vi "Camera.vi"(0 "Camera in":refnum<class "Camera.lvclass">, 1 "Machine Vision":T4, 2 "Material":T3, 3 "Loop 0":bool, 5 "Stop":bool, 9 "BCG Image Processing":T2={"Brightness"=128.0, "Contrast"=45.0, "Gamma"=1.0} {"Brightness" scale=0.0..400.0; "Contrast" scale=0.0..90.0; "Gamma" scale=0.005..5.0}, 11 "error in (no error)":errorcluster, 12 "Camera settings":T1={"Gamma"=1.0, "Gain"=7, "Sharpness"=0, "Contrast"=0.009999999999999995, "Exposure"=0.0004073180282999787} {"Exposure" min=0.000244140625 max=0.5 scale=0.0002..0.5; "Contrast" min=0.0 max=1.0 scale=0.001..1.0; "Sharpness" min=0 max=2 step=1 scale=0.0..2.0; "Gain" min=0 max=100 step=1 scale=0.1..100.0; "Gamma" min=0.01 max=10.0 scale=0.01..10.0}, 14 "Override presets":bool) -> (4 "Camera out":refnum<class "Camera.lvclass">, 6 "Average Strength":dbl, 8 "Image":T5(plugin-control), 10 "Camera":dbl[](array[numeric]), 13 "Radius (Real-World)":dbl, 15 "error out":errorcluster)   [LabVIEW 2020, in "Camera.lvclass"]
uses:
  Camera.lvclass
  Machine Vision.ctl
  Material.ctl
  Image processing.ctl
  Camera settings.ctl
  <vilib>/vision/NI_Vision_Development_Module.lvlib
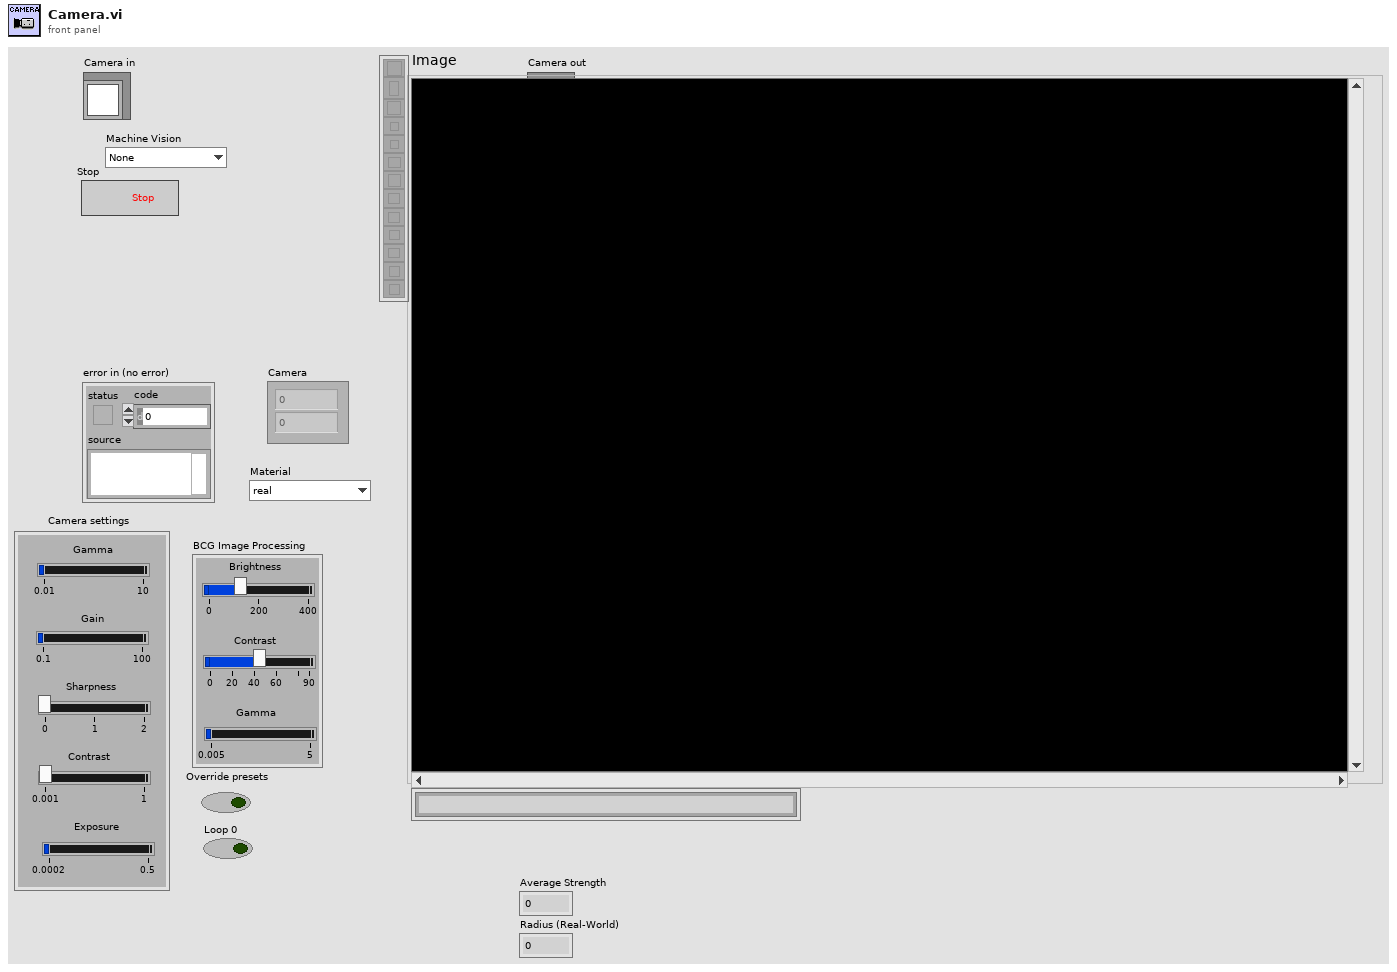
[diagram p1: front panel]
types:
  T1 = typedef "Camera.lvclass/Camera settings.ctl" = cluster{"Gamma":dbl, "Gain":i64, "Sharpness":i64, "Contrast":dbl, "Exposure":dbl}
  T2 = typedef "Camera.lvclass/Image processing.ctl" = cluster{"Brightness":sgl, "Contrast":sgl, "Gamma":sgl}
  T3 = typedef "Camera.lvclass/Material.ctl" = enum16{"real", "dummy", "PETG"}
  T4 = typedef "Camera.lvclass/Machine Vision.ctl" = enum16{"None", "Tray Fiducials", "HPK Silicon", "100um dot", "Hexaboard", "Corner (TL, BR)", "Corner (BL, TR)"}
  T5 = typedef "IMAQ Image.ctl" = refnum<image>
  T6 = cluster{"Center (Pixels)":cluster{"X":sgl, "Y":sgl}, "Radius (Pixels)":dbl, "Center (Real-World)":cluster{"X":sgl, "Y":sgl}, "Radius (Real-World)":dbl, "Roundness (Real-World)":dbl, "Average Strength":dbl, "Average SNR (dB)":dbl}
  T7 = cluster{"output string":sgl, "output string":sgl}
  T8 = typedef "ROI Descriptor" = cluster{"Global Rectangle":i32[], "Contours":cluster{"ID":enum32{"External", "Internal"}, "Type":u32, "Coordinates":i32[]}[]}
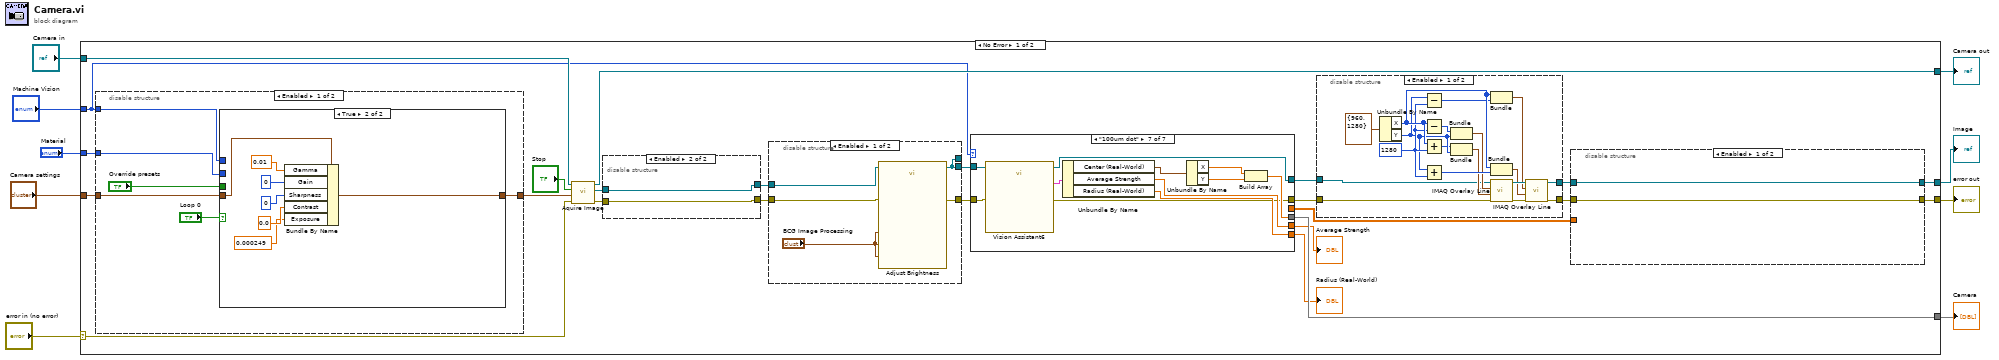
[diagram p0: block diagram]
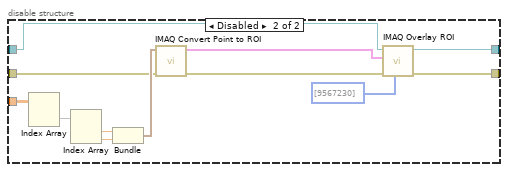
[diagram p2: hidden frame]
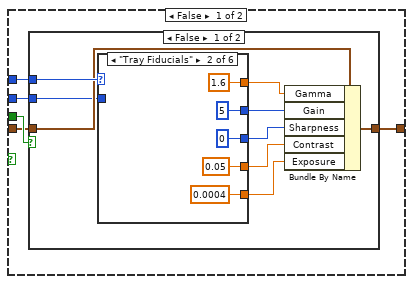
[diagram p5: hidden frame]
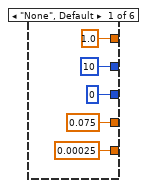
[diagram p6: hidden frame]
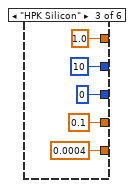
[diagram p7: hidden frame]
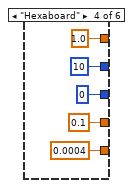
[diagram p8: hidden frame]
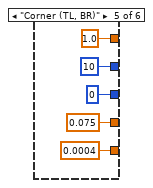
[diagram p9: hidden frame]
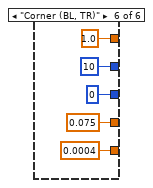
[diagram p10: hidden frame]
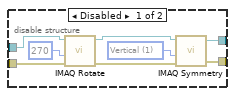
[diagram p13: hidden frame]
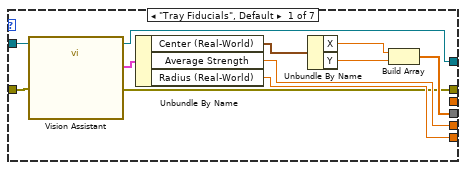
[diagram p14: hidden frame]
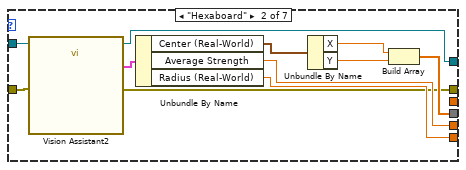
[diagram p15: hidden frame]
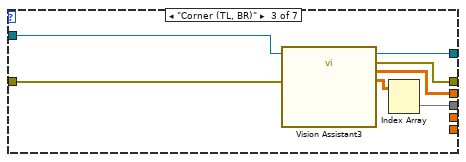
[diagram p16: hidden frame]
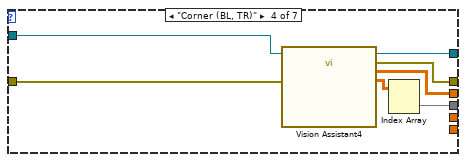
[diagram p17: hidden frame]
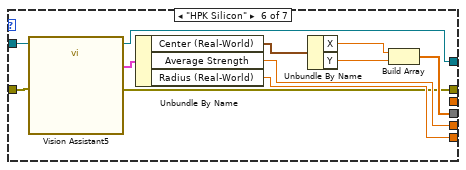
[diagram p19: hidden frame]
diagram:
  n1 = case shown="No Error" "error in (no error)" {
    selector: "error in (no error)" -> [w16 w205]
    tunnel: [w10 w205] -> w8
    tunnel: [w31 w204] -> w7
    tunnel: "Camera in" -> [w32 w204]
    tunnel: [w30 _] -> w5
    tunnel: [w20 _] -> w4
    tunnel: "Machine Vision" -> [w26 _]
    tunnel: "Camera settings" -> [w27 _]
    tunnel: "Material" -> [w25 _]
    frame No Error {
      n2 = disable-structure shown="Enabled" {
        disable-tunnel: w26 -> [w80 _]
        disable-tunnel: w27 -> [w79 w133]
        disable-tunnel: [w78 w133] -> w28
        disable-tunnel: w25 -> [w75 _]
        frame Enabled {
          n3 = case shown="True" "Loop 0" {
            tunnel: "Override presets" -> [w85 _]
            tunnel: w80 -> [w84 _]
            tunnel: w79 -> [w83 w132]
            tunnel: [w82 w131] -> w78
            tunnel: w75 -> [w81 _]
            frame False {
              n4 = case shown="False" w85 {
                tunnel: w84 -> [w94 _]
                tunnel: w83 -> [w93 w125]
                tunnel: [w87 w125] -> w82
                tunnel: w81 -> [w86 _]
                frame False {
                  n5 = case shown="\"Tray Fiducials\"" w94 {
                    tunnel: [1.0 ("Gamma::Value") 1.6 ("Gamma::Value") 1.0 ("Gamma::Value") 1.0 ("Gamma::Value") 1.0 ("Gamma::Value") 1.0 ("Gamma::Value")] -> w92
                    tunnel: [i64 10 ("Gain::Value") i64 5 ("Gain::Value") i64 10 ("Gain::Value") i64 10 ("Gain::Value") i64 10 ("Gain::Value") i64 10 ("Gain::Value")] -> w91
                    tunnel: [i64 0 ("Sharpness::Value") i64 0 ("Sharpness::Value") i64 0 ("Sharpness::Value") i64 0 ("Sharpness::Value") i64 0 ("Sharpness::Value") i64 0 ("Sharpness::Value")] -> w90
                    tunnel: [0.075 ("Contrast::Value") 0.05 ("Contrast::Value") 0.1 ("Contrast::Value") 0.1 ("Contrast::Value") 0.075 ("Contrast::Value") 0.075 ("Contrast::Value")] -> w89
                    tunnel: [0.00025 ("Exposure::Value") 0.0004 ("Exposure::Value") 0.0004 ("Exposure::Value") 0.0004 ("Exposure::Value") 0.0004 ("Exposure::Value") 0.0004 ("Exposure::Value")] -> w88
                    tunnel: w86 -> [_ _ _ _ _ _]
                    frame "None", Default {
                    }
                    frame "Tray Fiducials" {
                    }
                    frame "HPK Silicon" {
                    }
                    frame "Hexaboard" {
                    }
                    frame "Corner (TL, BR)" {
                    }
                    frame "Corner (BL, TR)" {
                    }
                  }
                  n6 = Bundle By Name(cluster=w93, "Gamma"=w92, "Gain"=w91, "Sharpness"=w90, "Contrast"=w89, "Exposure"=w88) -> (w87:T1)
                }
                frame True {
                }
              }
            }
            frame True {
              n7 = Bundle By Name(cluster=w132, "Gamma"=0.01, "Gain"=i64 0, "Sharpness"=i64 0, "Contrast"=0.0, "Exposure"=0.000249) -> (w131:T1)
            }
          }
        }
        frame Disabled {
        }
      }
      n8 = call-dynamic "Aquire Image.vi"("error in (no error)"=w16, "Cluster"=w28, "Stop"="Stop", "Camera in"=w32) -> ("error out"=w15:errorcluster, "Image Out"=w29:T5, "Camera out"=w31:refnum<class "Camera.lvclass">)  [unwired: 5 in]
      n9 = disable-structure shown="Enabled" {
        disable-tunnel: w29 -> [w140 w143]
        disable-tunnel: [w139 w143] -> w24
        disable-tunnel: w15 -> [w136 w142]
        disable-tunnel: [w134 w142] -> w14
        frame Disabled {
          w138 = u32 1 items=["Horizontal", "Vertical", "Central", "1st Diagonal", "2nd Diagonal"] ("Type of Symmetry")
          n10 = call "IMAQ Rotate"("error in (no error)"=w136, "Angle (degrees)"=270, "Image Src"=w140) -> ("error out"=w135:errorcluster, "Image Dst Out"=w137:T5)  [unwired: 7 in]
          n11 = call "IMAQ Symmetry"("error in (no error)"=w135, "Type of Symmetry"=w138, "Image Src"=w137) -> ("error out"=w134:errorcluster, "Image Dst Out"=w139:T5)  [unwired: 2 in]
        }
        frame Enabled {
        }
      }
      n12 = disable-structure shown="Enabled" {
        disable-tunnel: w24 -> [w72 w74]
        disable-tunnel: [w70 w74] -> _
        disable-tunnel: [w70 _] -> w23
        disable-tunnel: w14 -> [w69 w73]
        disable-tunnel: [w68 w73] -> w13
        frame Enabled {
          n13 = call "Adjust Brightness"("Image In"=w72, "Red BCG Values (Brightness 1)"="BCG Image Processing", "Green BCG Values (Brightness 1)"="BCG Image Processing", "Blue BCG Values (Brightness 1)"="BCG Image Processing", "error in"=w69) -> ("Image Out"=w70:T5, "error out"=w68:errorcluster)  [unwired: 21 in]
        }
        frame Disabled {
        }
      }
      n14 = case shown="\"100um dot\"" w26 {
        tunnel: [w148 w160 w170 w177 _ w188 w199] -> w30
        tunnel: [w150 w161 w172 w179 w181 w189 w200] -> w22
        tunnel: w23 -> [w151 w159 w169 w176 w181 w186 w197]
        tunnel: [w146 w157 _ _ _ w185 w196] -> w19
        tunnel: [w147 w158 _ _ _ w184 w195] -> w18
        tunnel: [_ _ w168 w175 _ _ _] -> w17
        tunnel: w13 -> [w145 w155 w167 w174 w180 w183 w194]
        tunnel: [w144 w156 w166 w173 w180 w182 w193] -> w12
        frame "Tray Fiducials", Default {
          n15 = call "Vision Assistant"("Image In"=w151, "error in"=w145) -> ("Image Out"=w150:T5, "Fitted Circle (Find Circular Edge 1)"=w149:T6, "error out"=w144:errorcluster)  [unwired: 23 in]
          n16 = Unbundle By Name(w149) -> ("Center (Real-World)"=w152:cluster{"X":sgl, "Y":sgl}, "Average Strength"=w147:dbl, "Radius (Real-World)"=w146:dbl)
          n17 = Unbundle By Name(w152) -> ("X"=w154:sgl, "Y"=w153:sgl)
          n18 = Build Array(w154, w153) -> (w148:sgl[])
        }
        frame "Hexaboard" {
          n19 = call "Vision Assistant2"("Image In"=w159, "error in"=w155) -> ("Image Out"=w161:T5, "Fitted Circle (Find Circular Edge 1)"=w163:T6, "error out"=w156:errorcluster)  [unwired: 23 in]
          n20 = Unbundle By Name(w163) -> ("Center (Real-World)"=w165:cluster{"X":sgl, "Y":sgl}, "Average Strength"=w158:dbl, "Radius (Real-World)"=w157:dbl)
          n21 = Unbundle By Name(w165) -> ("X"=w164:sgl, "Y"=w162:sgl)
          n22 = Build Array(w164, w162) -> (w160:sgl[])
        }
        frame "Corner (TL, BR)" {
          n23 = call "Vision Assistant3"("Image In"=w169, "error in"=w167) -> ("Image Out"=w172:T5, "error out"=w166:errorcluster, "Caliper Results (Top Left, Bottom Right)"=w168:sgl[][], "Calibrated Results (Top Left, Bottom Right)"=w171:sgl[][])  [unwired: 22 in]
          n24 = Index Array(array=w171) -> (element=w170:sgl[])  [unwired: 2 in]
        }
        frame "Corner (BL, TR)" {
          n25 = call "Vision Assistant4"("Image In"=w176, "error in"=w174) -> ("Image Out"=w179:T5, "error out"=w173:errorcluster, "Caliper Results (Bottom Left, Top Right)"=w175:sgl[][], "Calibrated Results (Bottom Left, Top Right)"=w178:sgl[][])  [unwired: 22 in]
          n26 = Index Array(array=w178) -> (element=w177:sgl[])  [unwired: 2 in]
        }
        frame "None" {
        }
        frame "HPK Silicon" {
          n27 = call "Vision Assistant5"("Image In"=w186, "error in"=w183) -> ("Image Out"=w189:T5, "Fitted Circle (Find Circular Edge 1)"=w187:T6, "error out"=w182:errorcluster)  [unwired: 23 in]
          n28 = Unbundle By Name(w187) -> ("Center (Real-World)"=w192:cluster{"X":sgl, "Y":sgl}, "Average Strength"=w184:dbl, "Radius (Real-World)"=w185:dbl)
          n29 = Unbundle By Name(w192) -> ("X"=w191:sgl, "Y"=w190:sgl)
          n30 = Build Array(w191, w190) -> (w188:sgl[])
        }
        frame "100um dot" {
          n31 = call "Vision Assistant6"("Image In"=w197, "error in"=w194) -> ("Image Out"=w200:T5, "Fitted Circle (Find Circular Edge 1)"=w198:T6, "error out"=w193:errorcluster)  [unwired: 23 in]
          n32 = Unbundle By Name(w198) -> ("Center (Real-World)"=w203:cluster{"X":sgl, "Y":sgl}, "Average Strength"=w195:dbl, "Radius (Real-World)"=w196:dbl)
          n33 = Unbundle By Name(w203) -> ("X"=w202:sgl, "Y"=w201:sgl)
          n34 = Build Array(w202, w201) -> (w199:sgl[])
        }
      }
      "Radius (Real-World)" <- w19
      "Average Strength" <- w18
      n35 = disable-structure shown="Enabled" {
        disable-tunnel: w22 -> [w52 w67]
        disable-tunnel: [w51 w67] -> w21
        disable-tunnel: w12 -> [w50 w66]
        disable-tunnel: [w48 w66] -> w11
        frame Enabled {
          w59 = 1280
          n36 = Unbundle By Name(cluster{"X":i32, "Y":i32} {"X"=960, "Y"=1280} ("Cross Hair coordinates")) -> ("X"=w62:i32, "Y"=w58:i32)
          n37 = Subtract(x=w58, y=w59) -> (x-y=w60:i32)
          n38 = Subtract(x=w62, y=w59) -> (x-y=w54:i32)
          n39 = Add(x=w62, y=w59) -> (x+y=w55:i32)
          n40 = Add(x=w58, y=w59) -> (x+y=w61:i32)
          n41 = Bundle(w54, "Y"=w58) -> (w57:cluster{i32, "Y":i32})  [unwired: 1 in]
          n42 = Bundle(w55, "Y"=w58) -> (w56:cluster{i32, "Y":i32})  [unwired: 1 in]
          n43 = Bundle("X"=w62, w60) -> (w63:cluster{"X":i32, i32})  [unwired: 1 in]
          n44 = Bundle("X"=w62, w61) -> (w64:cluster{"X":i32, i32})  [unwired: 1 in]
          n45 = call "IMAQ Overlay Line"("error in (no error)"=w50, "End Point"=w56, "Start Point"=w57, "Image"=w52) -> ("error out"=w49:errorcluster, "Image Out"=w65:T5)  [unwired: 6 in]
          n46 = call "IMAQ Overlay Line"("error in (no error)"=w49, "End Point"=w64, "Start Point"=w63, "Image"=w65) -> ("error out"=w48:errorcluster, "Image Out"=w51:T5)  [unwired: 6 in]
        }
        frame Disabled {
        }
      }
      n47 = disable-structure shown="Enabled" {
        disable-tunnel: [w35 w43] -> w20
        disable-tunnel: w21 -> [w35 w42]
        disable-tunnel: w17 -> [_ w41]
        disable-tunnel: w11 -> [w34 w38]
        disable-tunnel: [w34 w36] -> w10
        frame Enabled {
        }
        frame Disabled {
          n48 = Index Array(array=w41) -> (element=w40:sgl[])  [unwired: 2 in]
          n49 = Index Array(array=w40) -> (element #1=w44:sgl, element #2=w46:sgl)  [unwired: 2 in]
          n50 = Bundle("output string"=w44, "output string"=w46) -> (w47:T7)  [unwired: 1 in]
          n51 = call "IMAQ Convert Point to ROI"("error in (no error)"=w38, "Point"=w47) -> ("error out"=w37:errorcluster, "ROI Descriptor"=w45:T8)  [unwired: 7 in]
          n52 = call "IMAQ Overlay ROI"("Colors (Green)"=u32[] [9567230], "error in (no error)"=w37, "ROI Descriptor"=w45, "Image"=w42) -> ("error out"=w36:errorcluster, "Image Out"=w43:T5)  [unwired: 6 in]
        }
      }
    }
    frame Error {
    }
  }
  "error out" <- w8
  "Camera out" <- w7
  "Camera" <- w5
  "Image" <- w4
